vi "Main.vi"(8 "error in (no error)":errorcluster, 11 "Logging Thread in":refnum<class "Logging Thread.lvclass">) -> (0 "error out":errorcluster, 3 "Logging Thread out":refnum<class "Logging Thread.lvclass">)   [LabVIEW 2017, in "DSF Core.lvlib" / "Logging Thread.lvclass"]
uses:
  Logging Thread.lvclass
  Thread.lvclass
  C:/Git/DSF/Core/Classes/Thread/Thread.lvclass
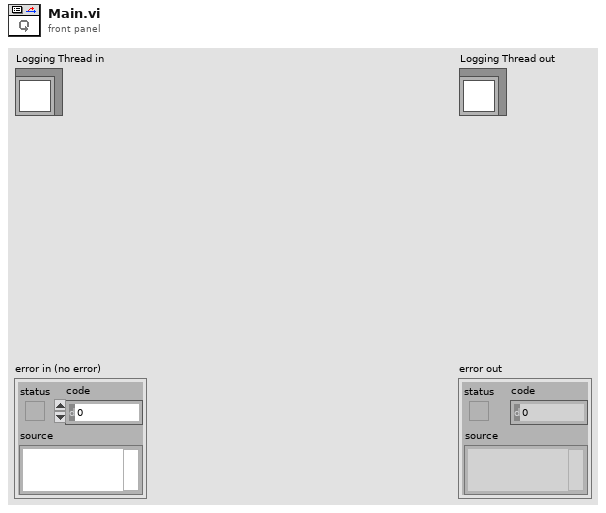
[diagram p1: front panel]
types:
  T1 = typedef "DSF Core.lvlib/Logging Interface.lvclass/Command Data.ctl" = cluster{"Command":T2, "Parameters":T3}
  T2 = typedef "DSF Core.lvlib/Logging Interface.lvclass/Command.ctl" = enum8{"Idle", "Start", "Log Framework State", "Log Plugin State", "Log Dispatcher State", "Shutdown"}
  T3 = typedef "DSF Core.lvlib/Logging Interface.lvclass/Parameters.ctl" = cluster{"arg1":u64, "arg2":u64}
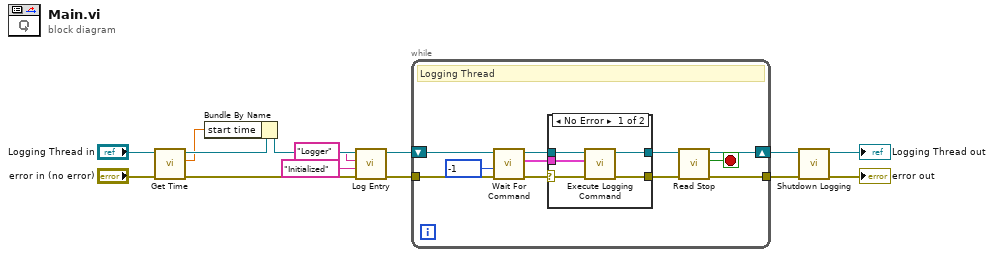
[diagram p0: block diagram]
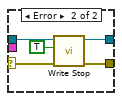
[diagram p2: hidden frame]
diagram:
  n1 = call "Get Time.vi"("error in (no error)"="error in (no error)", "Logging Thread in"="Logging Thread in") -> ("error out"=w3:errorcluster, "time"=w7:dbl, "Logging Thread out"=w8:refnum<class "Logging Thread.lvclass">)  [unwired: 7 in]
  n2 = Bundle By Name(cluster=w8, "start time"=w7) -> (w5:refnum<class "Logging Thread.lvclass">)
  n3 = call "Log Entry.vi"("error in (no error)"=w3, "line text"="Initialized", "line tag"="Logger", "Logging Thread in"=w5) -> ("error out"=w2:errorcluster, "Logging Thread out"=w4:refnum<class "Logging Thread.lvclass">)  [unwired: 6 in]
  n4 = while {
    tunnel: w2 -> [w25]
    tunnel: [w17] -> w13
    shift-right: [w18] -> w14
    shift-left: w4 -> [w24]
    stop <- w16 stop-if-true
    # "Logging Thread"
    n5 = call "Wait For Command.vi"("error in (no error)"=w25, "timeout in ms (0)"=-1, "Logging Thread in"=w24) -> ("error out"=w23:errorcluster, "command"=w15:T1, "Logging Thread out"=w22:refnum<class "Logging Thread.lvclass">)  [unwired: 6 in]
    n6 = case shown="No Error" w23 {
      selector: w23 -> [w30 w33]
      tunnel: [w26 w31] -> w19
      tunnel: w22 -> [w29 w34]
      tunnel: [w27 w32] -> w20
      tunnel: w15 -> [w28 _]
      frame No Error {
        n7 = call "Execute Logging Command.vi"("error in (no error)"=w30, "command"=w28, "Logging Thread in"=w29) -> ("error out"=w26:errorcluster, "Logging Thread out"=w27:refnum<class "Logging Thread.lvclass">)  [unwired: 7 in]
      }
      frame Error {
        n8 = call "Write Stop.vi"("error in (no error)"=w33, "stop"=TRUE, "Thread in"=w34) -> ("error out"=w31:errorcluster, "Thread out"=w32:refnum<class "Logging Thread.lvclass">)  [unwired: 7 in]
      }
    }
    n9 = call "Read Stop.vi"("error in (no error)"=w19, "Thread in"=w20) -> ("error out"=w17:errorcluster, "stop"=w16:bool, "Thread out"=w18:refnum<class "Logging Thread.lvclass">)  [unwired: 7 in]
  }
  n10 = call "Shutdown Logging.vi"("error in (no error)"=w13, "Logging Thread in"=w14) -> ("error out"=→"error out":errorcluster, "Logging Thread out"=→"Logging Thread out":refnum<class "Logging Thread.lvclass">)  [unwired: 8 in]
